vi "Get Version.vi"(8 "error in (no error)":errorcluster, 11 "LabVIEW File in":refnum<class "LabVIEW File.lvclass">) -> (0 "error out":errorcluster, 3 "LabVIEW File out":refnum<class "LabVIEW File.lvclass">)   [LabVIEW 2020, in "Save for Previous Version.lvlib" / "LabVIEW File.lvclass"]
uses:
  LabVIEW File.lvclass
  \\Mac\Home/JKI/GitHub/save-for-previous-labview-version/source/File/File.lvclass/File.lvclass
  File/File.lvclass/File.lvclass/File.ctl
  LabVIEW File.lvclass/LabVIEW File.ctl
  File/File.lvclass/File.lvclass
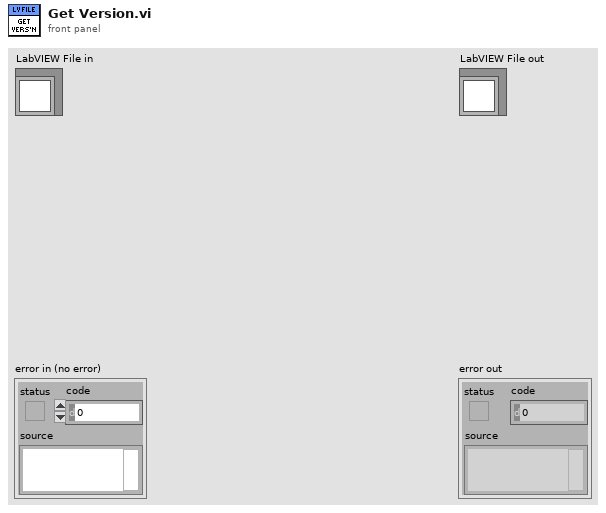
[diagram p1: front panel]
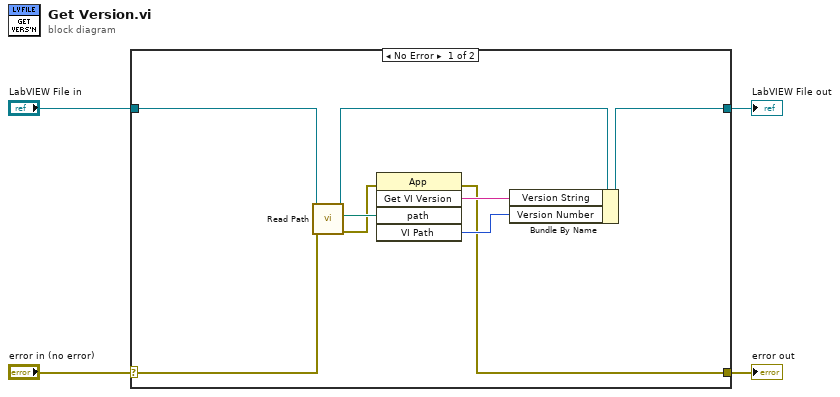
[diagram p0: block diagram]
diagram:
  n1 = case shown="No Error" "error in (no error)" {
    selector: "error in (no error)" -> [w9 w15]
    tunnel: [w10 w15] -> w3
    tunnel: [w5 w14] -> w1
    tunnel: "LabVIEW File in" -> [w7 w14]
    frame No Error {
      n2 = call "Read Path.vi"("error in (no error)"=w9, "File in"=w7) -> ("error out"=w8:errorcluster, "Path"=w13:path, "File out"=w6:refnum<class "LabVIEW File.lvclass">)  [unwired: 7 in]
      n3 = invoke class="App" method="Get VI Version"(error in=w8, "path"=w13) -> (error out=w10:errorcluster, "GetVIVers"=w12:string, "VI Path"=w11:u32)  [unwired: 3 in, 2 out]
      n4 = Bundle By Name(cluster=w6, "Version String"=w12, "Version Number"=w11) -> (w5:refnum<class "LabVIEW File.lvclass">)
    }
    frame Error {
    }
  }
  "error out" <- w3
  "LabVIEW File out" <- w1
